vi "PC Take Data No Objects.vi"(8 "error in (no error)":errorcluster, 11 "Photon Counter SR 400 in":T1={"Mode"=0, "Count Time"=0.0, "Trigger Frequency"=10000000.0, "Trigger External?"=FALSE, "Gate A Mode"=0, "Gate A Width"=0.0, "Gate A Delay"=0.0, "Gate B Mode"=0, "Gate B Width"=0.0, "Gate B Delay"=0.0} {"Mode" items=["A,B For T Preset", "A-B For T Preset", "A+B For T Preset", "A For B Preset"]; "Gate A Mode" items=["CW", "Fixed"]; "Gate B Mode" items=["CW", "Fixed"]}) -> (0 "error out":errorcluster, 1 "CPS B":dbl[unit], 2 "CPS A":dbl[unit], 3 "Photon counter SR 400 out":T1={"Mode"=0, "Count Time"=0.0, "Trigger Frequency"=10000000.0, "Trigger External?"=FALSE, "Gate A Mode"=0, "Gate A Width"=0.0, "Gate A Delay"=0.0, "Gate B Mode"=0, "Gate B Width"=0.0, "Gate B Delay"=0.0} {"Mode" items=["A,B For T Preset", "A-B For T Preset", "A+B For T Preset", "A For B Preset"]; "Gate A Mode" items=["CW", "Fixed"]; "Gate B Mode" items=["CW", "Fixed"]})   [LabVIEW 2012]
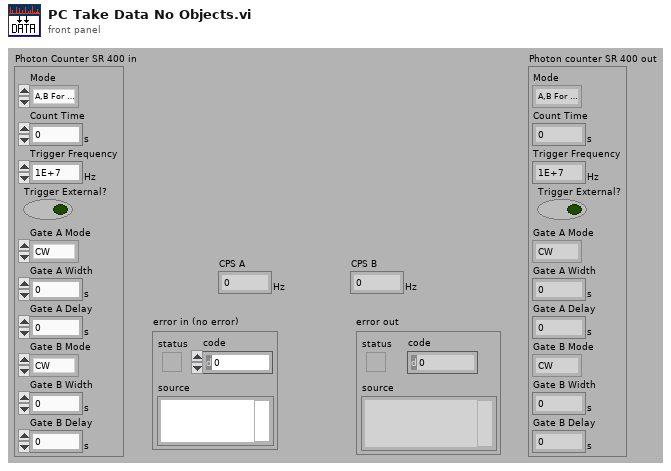
[diagram p1: front panel]
types:
  T1 = cluster{"Mode":u16, "Count Time":dbl[unit], "Trigger Frequency":dbl[unit], "Trigger External?":bool, "Gate A Mode":u16, "Gate A Width":dbl[unit], "Gate A Delay":dbl[unit], "Gate B Mode":u16, "Gate B Width":dbl[unit], "Gate B Delay":dbl[unit]}
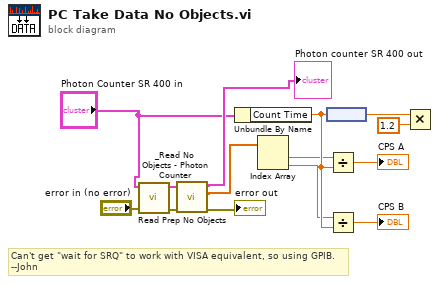
[diagram p0: block diagram]
diagram:
  # "Can't get \"wait for SRQ\" to work with VISA equivalent, so using GPIB. \n--John"
  n1 = call "Read Prep No Objects.vi"("error in (no error)"="error in (no error)", "Photon Counter SR 400 in"="Photon Counter SR 400 in") -> ("error out"=w3:errorcluster, "Photon Counter SR 400 out"=w2:T1)  [unwired: 8 in]
  n2 = call "_Read No Objects - Photon Counter.vi"("error in (no error)"=w3, "Photon Counter SR 400 in"=w2) -> ("error out"=→"error out":errorcluster, "4 Data Points"=w6:dbl[], "Photon Counter SR 400 out"=→"Photon counter SR 400 out":T1)  [unwired: 7 in]
  n3 = Unbundle By Name("Photon Counter SR 400 in") -> ("Count Time"=w14:dbl[unit])
  n4 = Index Array(array=w6) -> (element #1=w9:dbl, element #2=w8:dbl)  [unwired: 2 in]
  n5 = node(w14) -> (w12:dbl)
  n6 = Divide(x=w9, y=w14) -> (x/y=→"CPS A":dbl[unit])
  n7 = Divide(x=w8, y=w14) -> (x/y=→"CPS B":dbl[unit])
  n8 = Multiply(x=w12, y=1.2) -> ()  [unwired: 1 out]
